vi "Get Source Waveform Task Data.vi"(8 "error in (no error)":errorcluster, 11 "Task Item Ref":T1=18446744073709551615 format="%.0x") -> (0 "error out":errorcluster, 2 "Source Waveform Data":T2, 3 "Task Item Ref out":T1=18446744073709551615 format="%.0x")   [LabVIEW 2015, in "Waveform-Processing-Custom-Device System Explorer.lvlib"]
uses:
  Waveform-Processing-Custom-Device System Explorer.lvlib
  <vilib>/NI Veristand/Custom Device API/Custom Device Item Ref.ctl
  NationalInstruments.VeriStand.SystemStorage
  <vilib>/NI VeriStand/Custom Device API/Custom Device API.lvlib
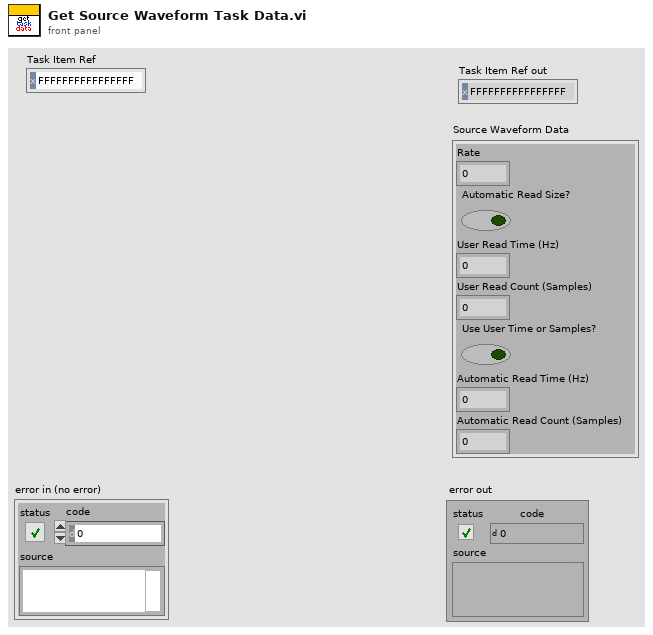
[diagram p1: front panel]
types:
  T1 = typedef "Custom Device API.lvlib/Custom Device Item Ref.ctl" = u64
  T2 = cluster{"Rate":dbl, "Automatic Read Size?":bool, "User Read Time (Hz) ":dbl, "User Read Count (Samples) ":u32, "Use User Time or Samples?":bool, "Automatic Read Time (Hz)":dbl, "Automatic Read Count (Samples)":u32}
  T3 = typedef "Custom Device API.lvlib/Custom Device Pointer.ctl" = refnum<k24>
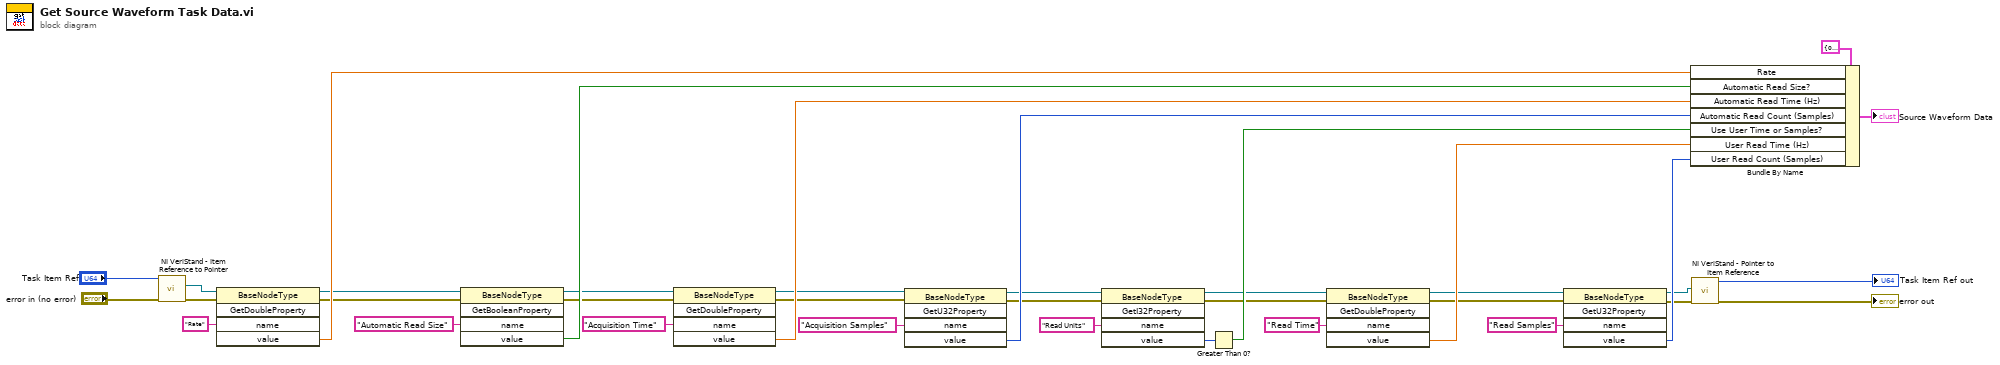
[diagram p0: block diagram]
diagram:
  n1 = call <vilib>:"NI VeriStand - Item Reference to Pointer.vi"("error in (no error)"="error in (no error)", "Item Ref in"="Task Item Ref") -> ("error out"=w34:errorcluster, "Node Pointer"=w35:T3)  [unwired: 6 in, 2 out]
  n2 = invoke class="BaseNodeType" method="GetDoubleProperty"(reference=w35, error in=w34, "name"="Rate") -> (reference out=w30:T3, error out=w29:errorcluster, "value"=w31:dbl)  [unwired: 2 in, 2 out]
  n3 = invoke class="BaseNodeType" method="GetBooleanProperty"(reference=w30, error in=w29, "name"="Automatic Read Size") -> (reference out=w25:T3, error out=w26:errorcluster, "value"=w27:bool)  [unwired: 2 in, 2 out]
  n4 = invoke class="BaseNodeType" method="GetDoubleProperty"(reference=w25, error in=w26, "name"="Acquisition Time") -> (reference out=w22:T3, error out=w21:errorcluster, "value"=w23:dbl)  [unwired: 2 in, 2 out]
  n5 = invoke class="BaseNodeType" method="GetU32Property"(reference=w22, error in=w21, "name"="Acquisition Samples") -> (reference out=w17:T3, error out=w18:errorcluster, "value"=w19:u32)  [unwired: 2 in, 2 out]
  n6 = invoke class="BaseNodeType" method="GetI32Property"(reference=w17, error in=w18, "name"="Read Units") -> (reference out=w12:T3, error out=w13:errorcluster, "value"=w15:i32)  [unwired: 2 in, 2 out]
  n7 = Greater Than 0?(x=w15) -> (x > 0?=w14:bool)
  n8 = invoke class="BaseNodeType" method="GetDoubleProperty"(reference=w12, error in=w13, "name"="Read Time") -> (reference out=w9:T3, error out=w8:errorcluster, "value"=w10:dbl)  [unwired: 2 in, 2 out]
  n9 = invoke class="BaseNodeType" method="GetU32Property"(reference=w9, error in=w8, "name"="Read Samples") -> (reference out=w3:T3, error out=w4:errorcluster, "value"=w6:u32)  [unwired: 2 in, 2 out]
  n10 = Bundle By Name(cluster=T2 {"Rate"=0.0, "Automatic Read Size?"=FALSE, "User Read Time (Hz) "=0.0, "User Read Count (Samples) "=0, "Use User Time or Samples?"=FALSE, "Automatic Read Time (Hz)"=0.0, "Automatic Read Count (Samples)"=0} ("Source Waveform Data"), "Rate"=w31, "Automatic Read Size?"=w27, "Automatic Read Time (Hz)"=w23, "Automatic Read Count (Samples)"=w19, "Use User Time or Samples?"=w14, "User Read Time (Hz)"=w10, "User Read Count (Samples)"=w6) -> (→"Source Waveform Data":T2)
  n11 = call <vilib>:"NI VeriStand - Pointer to Item Reference.vi"("error in (no error)"=w4, "Node Pointer"=w3) -> ("error out"=→"error out":errorcluster, "Item Ref out"=→"Task Item Ref out":T1)  [unwired: 8 in]
